vi "Sequence.AddDurationTrackingLoop.vi"(8 "error in (no error)":errorcluster, 9 "expressionString":string, 10 "Sequence Channels":T1, 11 ".NET Refnum in":refnum<k24>) -> (0 "error out":errorcluster, 3 ".NET Refnum out":refnum<k24>)   [LabVIEW 2015, in "Single Station Execution.lvlib"]
uses:
  Single Station Execution.lvlib
  NationalInstruments.VeriStand.RealTimeSequenceDefinitionApi
  Types/Compiled.SequenceChannels.ctl
  Types/Channel.Properties.ctl
  Main.Constants.vi
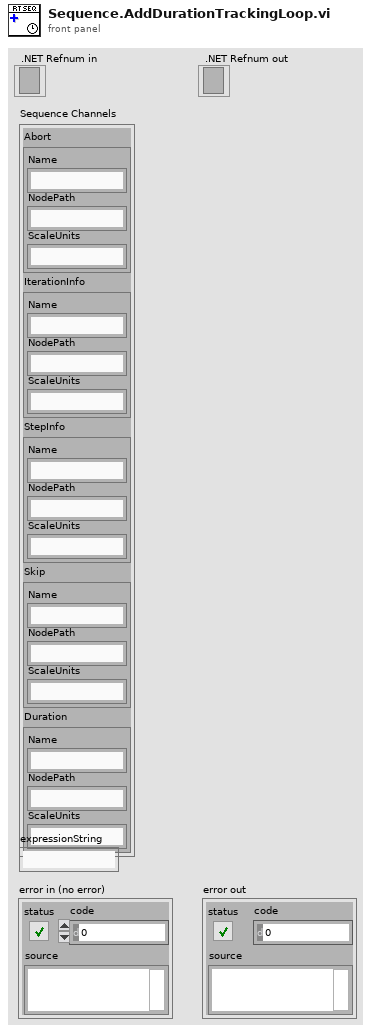
[diagram p1: front panel]
types:
  T1 = typedef "Single Station Execution.lvlib/Compiled.SequenceChannels.ctl" = cluster{"Abort":T2, "IterationInfo":T2, "StepInfo":T2, "Skip":T2, "Duration":T2}
  T2 = typedef "Single Station Execution.lvlib/Channel.Properties.ctl" = cluster{"Name":string, "NodePath":string, "ScaleUnits":string}
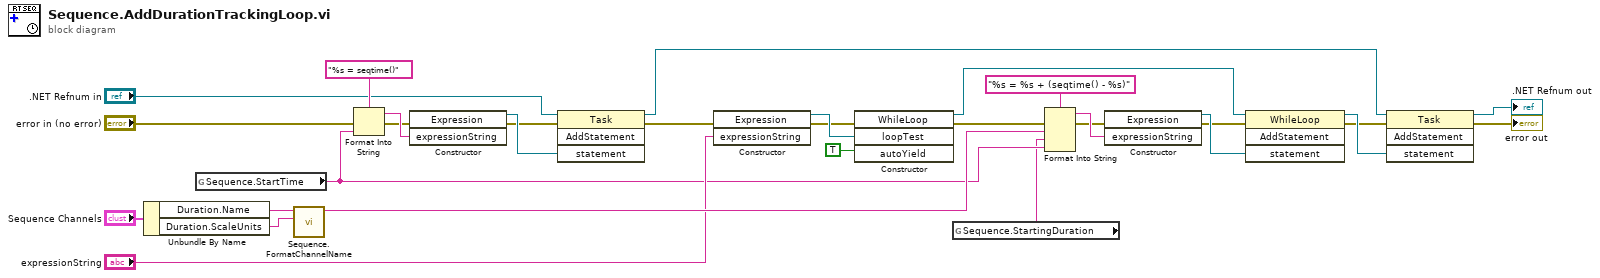
[diagram p0: block diagram]
diagram:
  n1 = Unbundle By Name("Sequence Channels") -> ("Duration.Name"=w28:string, "Duration.ScaleUnits"=w29:string)
  n2 = global read "Main.Constants.vi" "Sequence.StartTime"() -> (w2:string)
  n3 = call "Sequence.FormatChannelName.vi"("ScaleUnits"=w29, "Name"=w28) -> ("ChannelName"=w25:string)  [unwired: 9 in]
  n4 = Format Into String(format string="%s = seqtime()" ("expressionString"), error in="error in (no error)", w2) -> (resulting string=w24:string, error out=w22:errorcluster)  [unwired: 1 in]
  n5 = constructor class="Expression"(error in=w22, "expressionString"=w24) -> (reference out=w16:refnum<k24>, error out=w14:errorcluster)  [unwired: 2 in, 2 out]
  n6 = invoke class="Task" method="AddStatement"(reference=".NET Refnum in", error in=w14, "statement"=w16) -> (reference out=w19:refnum<k24>, error out=w15:errorcluster)  [unwired: 1 in, 2 out]
  n7 = constructor class="Expression"(error in=w15, "expressionString"="expressionString") -> (reference out=w5:refnum<k24>, error out=w4:errorcluster)  [unwired: 2 in, 2 out]
  n8 = constructor class="WhileLoop"(error in=w4, "loopTest"=w5, "autoYield"=TRUE) -> (reference out=w13:refnum<k24>, error out=w8:errorcluster)  [unwired: 2 in, 3 out]
  n9 = global read "Main.Constants.vi" "Sequence.StartingDuration"() -> (w1:string)
  n10 = Format Into String(format string="%s = %s + (seqtime() - %s)" ("expressionString"), error in=w8, w25, w1, w2) -> (resulting string=w10:string, error out=w9:errorcluster)  [unwired: 1 in]
  n11 = constructor class="Expression"(error in=w9, "expressionString"=w10) -> (reference out=w12:refnum<k24>, error out=w11:errorcluster)  [unwired: 2 in, 2 out]
  n12 = invoke class="WhileLoop" method="AddStatement"(reference=w13, error in=w11, "statement"=w12) -> (reference out=w20:refnum<k24>, error out=w18:errorcluster)  [unwired: 1 in, 2 out]
  n13 = invoke class="Task" method="AddStatement"(reference=w19, error in=w18, "statement"=w20) -> (reference out=→".NET Refnum out":refnum<k24>, error out=→"error out":errorcluster)  [unwired: 1 in, 2 out]
